vi "ExportImages.vi"(7 "output_directory":path, 8 "Transconductance..":refnum<vi>, 9 "Transconductance":refnum<vi>, 10 "Conductance..":refnum<vi>, 11 "Conductance":refnum<vi>) -> ()   [LabVIEW 2016]
panel:
  out "appended path 4":path
  out "appended path 3":path
  out "appended path 2":path
  out "appended path":path
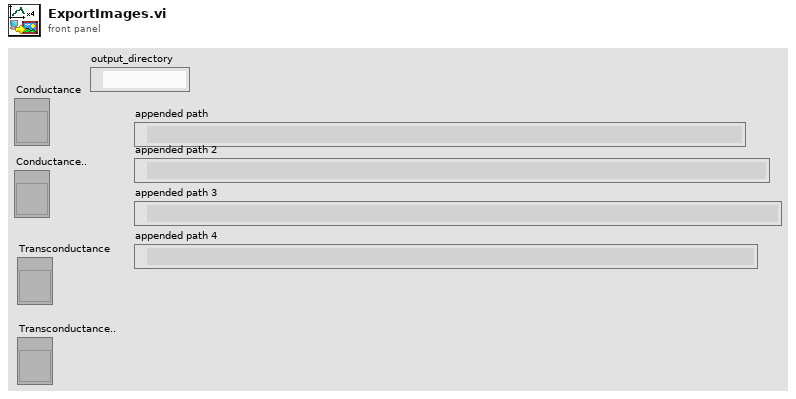
[diagram p1: front panel]
types:
  T1 = typedef "imagedata.ctl" = cluster{"image type":i32, "image depth":i32, "image":u8[], "mask":u8[], "colors":u32[], "Rectangle":cluster{"left":i16, "top":i16, "right":i16, "bottom":i16}}
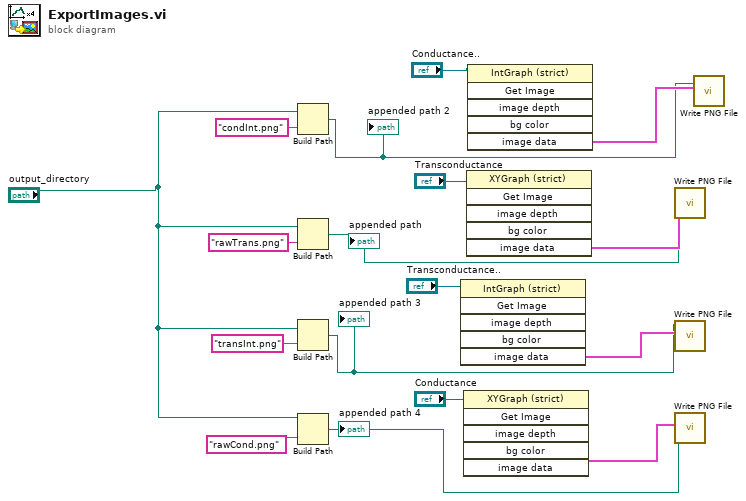
[diagram p0: block diagram]
diagram:
  n1 = Build Path(base path="output_directory", name or relative path="condInt.png") -> (appended path=w13:path)
  "appended path 2" <- w13
  n2 = Build Path(base path="output_directory", name or relative path="rawTrans.png") -> (appended path=w9:path)
  "appended path" <- w9
  n3 = Build Path(base path="output_directory", name or relative path="transInt.png") -> (appended path=w12:path)
  "appended path 3" <- w12
  n4 = Build Path(base path="output_directory", name or relative path="rawCond.png") -> (appended path=w8:path)
  "appended path 4" <- w8
  n5 = invoke class="IntGraph (strict)" method="Get Image"(reference="Transconductance..") -> ("image data"=w15:T1)  [unwired: 5 in, 5 out]
  n6 = invoke class="XYGraph (strict)" method="Get Image"(reference="Conductance") -> ("image data"=w11:T1)  [unwired: 5 in, 5 out]
  n7 = invoke class="XYGraph (strict)" method="Get Image"(reference="Transconductance") -> ("image data"=w10:T1)  [unwired: 5 in, 5 out]
  n8 = invoke class="IntGraph (strict)" method="Get Image"(reference="Conductance..") -> ("image data"=w17:T1)  [unwired: 5 in, 5 out]
  n9 = call <vilib>:"Write PNG File.vi"("image data"=w10, "path to PNG file"=w9) -> ()  [unwired: 8 in, 2 out]
  n10 = call <vilib>:"Write PNG File.vi"("image data"=w15, "path to PNG file"=w12) -> ()  [unwired: 8 in, 2 out]
  n11 = call <vilib>:"Write PNG File.vi"("image data"=w11, "path to PNG file"=w8) -> ()  [unwired: 8 in, 2 out]
  n12 = call <vilib>:"Write PNG File.vi"("image data"=w17, "path to PNG file"=w13) -> ()  [unwired: 8 in, 2 out]
